vi "Self-Test.vi"(8 "error in (no error)":errorcluster {"code" format="%.0x"}, 11 "instrument handle":refnum<k15>) -> (0 "error out":errorcluster {"code" format="%.0x"}, 1 "self-test message":string, 2 "self test result":i16 format="%.0g", 3 "instrument handle out":refnum<k15>)   [LabVIEW 2014, in "Agilent NA.lvlib"]
doc: "Performs an instrument self test, waits for the instrument to complete the test, and queries the instrument for the results. If the instrument passes the test, TestResult is zero and TestMessage is 'Self test passed'."
uses:
  Agilent NA.lvlib
  AgNA.dll
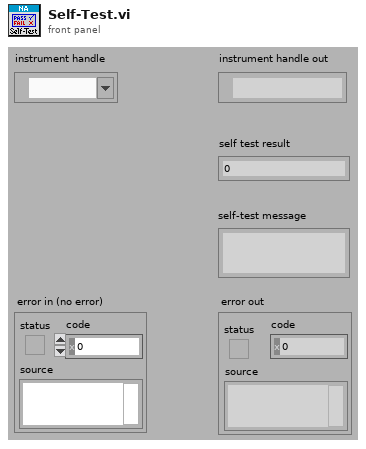
[diagram p1: front panel]
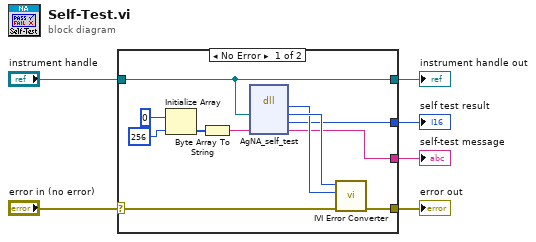
[diagram p0: block diagram]
diagram:
  n1 = case shown="No Error" "error in (no error)" {
    selector: "error in (no error)" -> [w9 w19]
    tunnel: [w13 w19] -> w6
    tunnel: [w10 w18] -> w5
    tunnel: "instrument handle" -> [w10 w18]
    tunnel: [w8 _] -> w2
    tunnel: [w7 _] -> w1
    frame No Error {
      n2 = Initialize Array(u8 0, 256) -> (w16:u8[])
      n3 = Byte Array To String(unsigned byte array=w16) -> (string=w15:string)
      n4 = dll-call lib="AgNA**.dll" fn="AgNA_self_test" ("LabVIEW:IviDmm_self_test")("instrument handle"=w10, "self-test message"=w15) -> ("Status"=w12:i32, "instrument handle"=w14:u32, "self test result"=w8:i16, "self-test message"=w7:string)  [unwired: 3 in, 3 out]
      n5 = call "IVI Error Converter.vi"("error in (no error)"=w9, "IVI error code (0)"=w12, "instrument handle"=w14) -> ("error out"=w13:errorcluster)  [unwired: 7 in, 1 out]
    }
    frame Error {
    }
  }
  "error out" <- w6
  "instrument handle out" <- w5
  "self test result" <- w2
  "self-test message" <- w1
